vi "BindCtrlEvent.vi"(1 "Stop":refnum<vi>, 2 "VI":refnum<vi>, 3 "Data":variant, 4 "Type":T1=enum."Value Change", 5 "Ctrl":refnum<vi>, 6 "Name":string) -> (0 "Event":refnum<event-registration>)   [LabVIEW 2014]
uses:
  <vilib>/event_ctls.llb/lveventtype.ctl
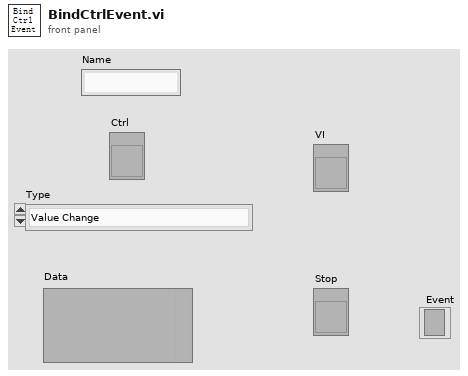
[diagram p1: front panel]
types:
  T1 = typedef "lveventtype.ctl" = enum32{"Null", "Timeout", "Annotation Menu Selection", "Annotation Menu Selection?", "App Instance Close", "App Instance Close?", "Autoscale Range Change", "Bookmark Info Change", "Cell Edit", "Cell Edit?", "Cursor Grab", "Cursor Grab?", "Cursor Menu Selection", "Cursor Menu Selection?", "Cursor Move", "Cursor Release", "Data Change", "Direction Change", "Display State Change", "Drag Ended", "Drag Enter", "Drag Leave", "Drag Over", "Drag Source Update", "Drag Starting", "Drag Starting?", "Drop", "Exec State Change", "Key Down", "Key Down?", "Key Repeat", "Key Repeat?", "Key Up", "Listbox Double Click", "Menu Activation?", "Menu Selection (App)", "Menu Selection? (App)", "Menu Selection (User)", "Mouse Down", "Mouse Down?", "Mouse Enter", "Mouse Leave", "Mouse Move", "Mouse Up", "Mouse Wheel", "NI Security User Change (App)", "Pane Size", "Panel Close", "Panel Close?", "Panel Resize", "Plot Attribute Change", "Scale Range Change", "Shortcut Menu Activation?", "Shortcut Menu Selection (App)", "Shortcut Menu Selection? (App)", "Shortcut Menu Selection (User)", "Tree Double Click", "Tree Drag", "Tree Drag?", "Tree Drop", "Tree Drop?", "Tree Item Close", "Tree Item Close?", "Tree Item Open", "Tree Item Open?", "User Event", "Value Change"}
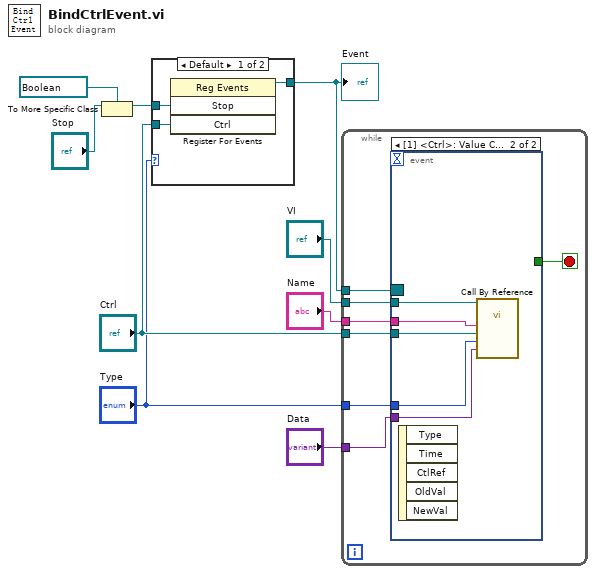
[diagram p0: block diagram]
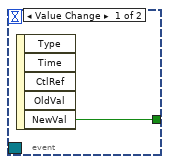
[diagram p2: hidden frame]
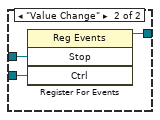
[diagram p3: hidden frame]
diagram:
  n1 = To More Specific Class(target class=refnum<vi> refnum ("Stop"), reference="Stop") -> (specific class reference=w3:refnum<vi>)  [unwired: 1 in, 1 out]
  n2 = case shown="Default" "Type" {
    tunnel: "Ctrl" -> [w11 w14]
    tunnel: w3 -> [w12 w15]
    tunnel: [w10 w13] -> w6
    frame Default {
      n3 = register-events(w12, w11) -> (reference out=w10:refnum<event-registration>)  [unwired: 2 in, 1 out]
    }
    frame "Value Change" {
      n4 = register-events(w15, w14) -> (reference out=w13:refnum<event-registration>)  [unwired: 2 in, 1 out]
    }
  }
  "Event" <- w6
  n5 = while {
    tunnel: "Ctrl" -> [w22]
    tunnel: "Type" -> [w21]
    tunnel: "Data" -> [w20]
    tunnel: w6 -> [w19]
    tunnel: "Name" -> [w17]
    tunnel: "VI" -> [w16]
    stop <- w18 stop-if-true
    n6 = event shown="[1] <Ctrl>: Value Change" {
      selector: w19 -> [_ _]
      dyn-events: _ -> [_ _]
      timeout: _ -> [_ _]
      tunnel: w22 -> [_ w28]
      tunnel: w21 -> [_ w27]
      tunnel: w20 -> [_ w26]
      tunnel: [w23 _] -> w18
      tunnel: w17 -> [_ w25]
      tunnel: w16 -> [_ w24]
      event Value Change {
        n7 = event-data() -> ("NewVal"=w23:bool)  [unwired: 1 in, 4 out]
      }
      event Value Change {
        n8 = event-data() -> ()  [unwired: 1 in, 5 out]
        n9 = call-by-ref "?"(reference=w24, "Data"=w26, "Type"=w27, "Ctrl"=w28, "Name"=w25) -> ()  [unwired: 1 in, 2 out]
      }
    }
  }
